vi "RB2 create post string DEMO.vi"() -> ()   [LabVIEW 2012]
panel:
  out "Post String":string
  out "Num Posts":i32
  in  "stop":bool
  out "error out":errorcluster
  in  "File Path":path
  out "Mars image":T1(plugin-control)
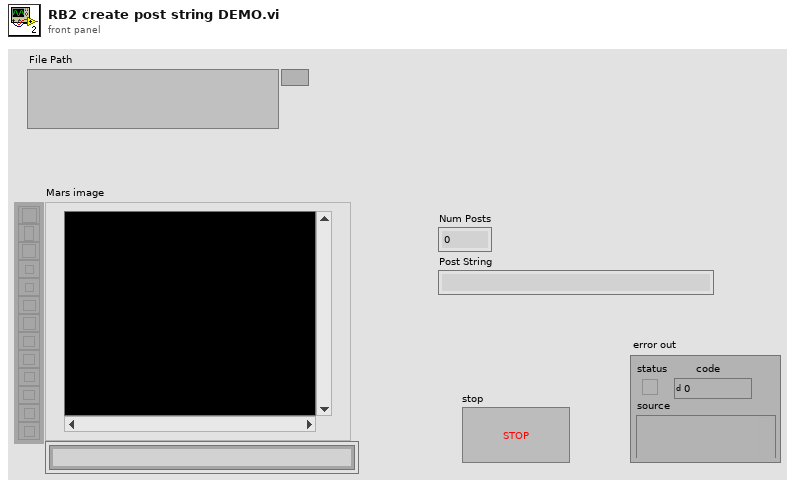
[diagram p1: front panel]
types:
  T1 = typedef "IMAQ Image.ctl" = refnum<image>
  T2 = typedef "Image Type" = u32
  T3 = cluster{"Pos. X":i32, "Pos. Y":i32, "Radius":i32, "Core Area":i32}[]
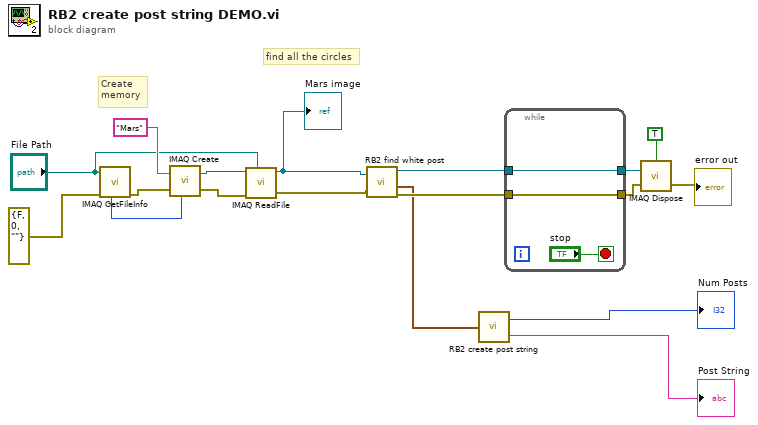
[diagram p0: block diagram]
diagram:
  # "find all the circles"
  # "Create \nmemory"
  n1 = call "IMAQ GetFileInfo"("error in (no error)"=errorcluster {"status"=FALSE, "code"=0, "source"=""}, "File Path"="File Path") -> ("error out"=w18:errorcluster, "Image Type"=w14:T2)  [unwired: 3 in, 5 out]
  n2 = call "IMAQ Create"("Image Name"="Mars", "Image Type"=w14, "error in (no error)"=w18) -> ("New Image"=w15:T1, "error out"=w16:errorcluster)  [unwired: 2 in]
  n3 = call "IMAQ ReadFile"("File Path"="File Path", "error in (no error)"=w16, "Image"=w15) -> ("error out"=w10:errorcluster, "Image Out"=w12:T1)  [unwired: 4 in, 3 out]
  "Mars image" <- w12
  n4 = call "RB2 find white post.vi"("Image In"=w12, "error in"=w10) -> ("Image Out"=w5:T1, "White dot\nLocation"=w3:T3, "error out"=w4:errorcluster)  [unwired: 1 out]
  n5 = call "RB2 create post string.vi"("White dot\nLocation"=w3) -> ("Num Posts"=→"Num Posts":i32, "Post String"=→"Post String":string)
  n6 = while {
    tunnel: w5 -> [w20]
    tunnel: w4 -> [w19]
    tunnel: [w20] -> w7
    tunnel: [w19] -> w6
    stop <- "stop" stop-if-true
  }
  n7 = call "IMAQ Dispose"("All Images? (No)"=TRUE, "Image"=w7, "error in (no error)"=w6) -> ("error out"=→"error out":errorcluster)  [unwired: 3 in]
